vi "Frequency_Response_Data_Smoothing_Shifting.vi"(0 "smoothing":bool, 1 "curveShifting":bool) -> ()   [LabVIEW 2012]
uses:
  <vilib>/Analysis/6fits.llb/Curve Fitting Criteria.ctl
  <vilib>/Analysis/6fits.llb/General Linear Fit Algorithm.ctl
  <vilib>/Analysis/NI_AALPro.lvlib
panel:
  in  "FG.FrequencyLists.FrequencyResponse_LimitLow.amplitude":dbl[](array[numeric])
  in  "FG.FrequencyLists.FrequencyResponse_LimitHigh.amplitude":dbl[](array[numeric])
  in  "Parameters.UUTResponseLevel.amplitude":dbl[](array[numeric])
  in  "Parameters.UUTResponseLevel.frequency":dbl[](array[numeric])
  in  "Parameters.RefAmplitude":dbl=0.357
  out "XY Graph 2":cluster{dbl[], dbl[]}[](graph)=[{[200.0, 212.0, 224.0, 236.0, 250.0, 265.0, 280.0, 300.0, 315.0, 335.0, 355.0, 375.0, 400.0, 425.0, 450.0, 475.0, 500.0, 530.0, 560.0, 600.0, 630.0, 670.0, 710.0, 750.0, 800.0, 850.0, 900.0, 950.0, 1000.0, 1060.0, 1120.0, 1180.0, 1250.0, 1320.0, 1400.0, 1500.0, 1600.0, 1700.0, 1800.0, 1900.0, 2000.0, 2120.0, 2240.0, 2360.0, 2500.0, 2650.0, 2800.0, 3000.0, 3150.0, 3350.0, 3750.0, 4000.0, 4250.0, 4500.0, 4750.0, 5000.0, 5300.0, 5600.0, 6000.0, 6300.0, 6700.0, 7100.0], [-7.2, -6.8, -6.3, -5.7, -5.9, -5.2, -5.2, -4.5, -4.4, -3.9, -3.4, -3.2, -2.9, -2.6, -2.4, -2.1, -1.9, -1.7, -1.5, -1.3, -1.3, -1.1, -0.8, -0.8, -0.7, -0.6, -0.3, -0.5, 0.0, -0.3, 0.0, 0.2, 0.2, 0.4, 0.8, 0.9, 1.5, 1.5, 1.6, 1.5, 1.4, 0.6, -0.5, -1.5, -1.6, -2.3, -2.5, -3.0, -2.7, -3.1, -4.1, -5.6, -4.3, -3.1, -2.0, -0.7, 0.0, -1.0, 0.0, 0.5, 0.9, 3.6]}, {[200.0, 212.0, 224.0, 236.0, 250.0, 265.0, 280.0, 300.0, 315.0, 335.0, 355.0, 375.0, 400.0, 425.0, 450.0, 475.0, 500.0, 530.0, 560.0, 600.0, 630.0, 670.0, 710.0, 750.0, 800.0, 850.0, 900.0, 950.0, 1000.0, 1060.0, 1120.0, 1180.0, 1250.0, 1320.0, 1400.0, 1500.0, 1600.0, 1700.0, 1800.0, 1900.0, 2000.0, 2120.0, 2240.0, 2360.0, 2500.0, 2650.0, 2800.0, 3000.0, 3150.0, 3350.0, 3750.0, 4000.0, 4250.0, 4500.0, 4750.0, 5000.0, 5300.0, 5600.0, 6000.0, 6300.0, 6700.0, 7100.0], [-1.1, -0.9, -0.8, -0.6, -0.4, -0.2, 0.0, 0.1, 0.3, 0.5, 0.7, 0.9, 1.0, 1.2, 1.3, 1.5, 1.6, 1.7, 1.9, 2.0, 2.2, 2.3, 2.5, 2.6, 2.8, 2.9, 3.0, 3.0, 3.0, 3.0, 3.1, 3.1, 3.2, 3.2, 3.3, 3.3, 3.4, 3.5, 3.5, 3.6, 3.6, 3.7, 3.8, 3.8, 3.9, 3.9, 4.0, 4.3, 4.7, 5.1, 5.5, 5.9, 6.2, 6.5, 6.8, 7.1, 7.4, 7.7, 8.0, 7.6, 7.2, 6.8]}, {[200.0, 212.0, 224.0, 236.0, 250.0, 265.0, 280.0, 300.0, 315.0, 335.0, 355.0, 375.0, 400.0, 425.0, 450.0, 475.0, 500.0, 530.0, 560.0, 600.0, 630.0, 670.0, 710.0, 750.0, 800.0, 850.0, 900.0, 950.0, 1000.0, 1060.0, 1120.0, 1180.0, 1250.0, 1320.0, 1400.0, 1500.0, 1600.0, 1700.0, 1800.0, 1900.0, 2000.0, 2120.0, 2240.0, 2360.0, 2500.0, 2650.0, 2800.0, 3000.0, 3150.0, 3350.0, 3750.0, 4000.0, 4250.0, 4500.0, 4750.0, 5000.0, 5300.0, 5600.0, 6000.0, 6300.0, 6700.0, 7100.0], [-12.1, -11.5, -10.9, -10.3, -9.7, -9.1, -8.5, -7.9, -7.3, -6.7, -6.1, -5.5, -5.0, -4.8, -4.7, -4.5, -4.4, -4.3, -4.1, -4.0, -3.8, -3.7, -3.5, -3.4, -3.2, -3.1, -3.0, -3.0, -3.0, -3.0, -3.0, -3.0, -3.0, -3.0, -3.0, -3.0, -3.0, -3.0, -3.0, -3.0, -3.0, -3.0, -3.0, -3.0, -3.0, -3.0, -3.0, -3.0, -3.0, -3.0, -3.0, -3.0, -3.0, -3.0, -3.0, -3.0, -3.0, -3.0, -3.0, -3.2, -3.4, -3.6]}, {[199.67341715670165, 211.21395804831343, 223.6398834792109, 236.91827495666882, 251.0357328679638, 265.996892987689, 281.82294298506883, 298.5501389312743, 316.2283218067368, 334.9194340084638, 354.69603585735297, 375.63982210550773, 397.84013844355104, 421.3924980079408, 446.39709788828463, 472.9573356346543, 501.1783257649011, 531.1654162719695, 563.0227051312137, 596.8515568077104, 632.7491189432191, 670.8070219208591, 711.1119966697486, 753.7490969501578, 798.8054485348823, 846.3740041392261, 896.5572983509842, 949.4712025604283, 1005.2486798902885, 1064.043540125737, 1126.0341946443743, 1191.4274113462093, 1260.4620695836447, 1333.4129150914612, 1410.594314916799, 1492.3640123491455, 1579.126881850313, 1671.3386839844277, 1769.50982034791, 1874.2090884994595, 1986.0674368900388, 2105.781688039848, 2234.1153513535733, 2371.8850498380257, 2519.936351237608, 2679.118589027189, 2850.2596824126886, 3034.140956331676, 3231.4719614539495, 3442.865294182133, 3668.8114166522637, 3909.6534767343846, 4165.562128033129, 4436.510349888317, 4722.248267375544, 5022.277971306764, 5335.8283382308855, 5661.829850434362, 5998.8894159417805, 6345.26518851645, 6698.841387660996, 7057.103118617942], [-6.65792244532346, -6.805075217908138, -6.694954533621337, -6.4014241964905665, -5.9867078721014835, -5.502234641802871, -4.989484556911629, -4.480834192917781, -4.000402203689442, -3.564894875677825, -3.184451682122225, -2.86349083725501, -2.6015548505066124, -2.394156080710522, -2.23362229030827, -2.1099421995544265, -2.0116110407215864, -1.9264761123053604, -1.842582333229369, -1.749017797050228, -1.636759285351931, -1.499476235935405, -1.3338989352742925, -1.139595038692343, -0.9186263930106383, -0.6752045532551799, -0.41534629936446726, -0.14652915289708227, 0.12265310626072844, 0.3828349231874647, 0.624223451218799, 0.8369430352399845, 1.0113796949782774, 1.1385256082953537, 1.2103235944797202, 1.2200115975391388, 1.1624671694930382, 1.0345519536649335, 0.8354561679748401, 0.5670430882316968, 0.23419353142577315, -0.15485086731731323, -0.5882549462370955, -1.0509038551327632, -1.5251194336044547, -1.9914149659351008, -2.4292499736703292, -2.8177850081983906, -3.1366364433300533, -3.366631267878519, -3.4905618782393444, -3.4939408709703432, -3.3657558353715027, -3.09922414606489, -2.69254775557457, -2.1496679869065165, -1.481020326128518, -0.7042892149500959, 0.15483715669758005, 1.0619120580818044, 1.972975425088389, 2.8337990676417735]}, {[200.0, 212.0, 224.0, 236.0, 250.0, 265.0, 280.0, 300.0, 315.0, 335.0, 355.0, 375.0, 400.0, 425.0, 450.0, 475.0, 500.0, 530.0, 560.0, 600.0, 630.0, 670.0, 710.0, 750.0, 800.0, 850.0, 900.0, 950.0, 1000.0, 1060.0, 1120.0, 1180.0, 1250.0, 1320.0, 1400.0, 1500.0, 1600.0, 1700.0, 1800.0, 1900.0, 2000.0, 2120.0, 2240.0, 2360.0, 2500.0, 2650.0, 2800.0, 3000.0, 3150.0, 3350.0, 3750.0, 4000.0, 4250.0, 4500.0, 4750.0, 5000.0, 5300.0, 5600.0, 6000.0, 6300.0, 6700.0, 7100.0], [-6.205157643136481, -6.020933720665548, -5.839820813498944, -5.661789291037467, -5.457941067757162, -5.244089074811557, -5.034895452852371, -4.763119446794431, -4.564576452219682, -4.306798833759117, -4.056840237791941, -3.814571221558727, -3.52235316631936, -3.2417019360107107, -2.9723725806568284, -2.7141230359897723, -2.4667141079946853, -2.1838004428542828, -1.9157540870861651, -1.5808002758181445, -1.3459098706888752, -1.0537598512323598, -0.7848342367946678, -0.5382573519035433, -0.2601588393533418, -0.014004002741201994, 0.20180170104589448, 0.3888108475350209, 0.548534539225186, 0.7062532479133133, 0.82925925924909, 0.919933372917582, 0.9879189654908209, 1.0185369247443874, 1.012085590476093, 0.9488508818517398, 0.8325442205002949, 0.6714424338723249, 0.4732695619414947, 0.24521268305773286, -0.00606226019973688, -0.3296005042348227, -0.668009124585811, -1.012545565513891, -1.4118853982716553, -1.8249503288668656, -2.211639742848497, -2.6702265839668047, -2.9619969125583223, -3.271384677495506, -3.591217499070522, -3.5837982599559837, -3.4242772734673714, -3.126780435781683, -2.7106446731240332, -2.198872448299305, -1.493935993511684, -0.7316998047271994, 0.3027856705332539, 1.048904055149677, 1.9656754194686528, 2.7927851528351084]}, {[200.0, 212.0, 224.0, 236.0, 250.0, 265.0, 280.0, 300.0, 315.0, 335.0, 355.0, 375.0, 400.0, 425.0, 450.0, 475.0, 500.0, 530.0, 560.0, 600.0, 630.0, 670.0, 710.0, 750.0, 800.0, 850.0, 900.0, 950.0, 1000.0, 1060.0, 1120.0, 1180.0, 1250.0, 1320.0, 1400.0, 1500.0, 1600.0, 1700.0, 1800.0, 1900.0, 2000.0, 2120.0, 2240.0, 2360.0, 2500.0, 2650.0, 2800.0, 3000.0, 3150.0, 3350.0, 3750.0, 4000.0, 4250.0, 4500.0, 4750.0, 5000.0, 5300.0, 5600.0, 6000.0, 6300.0, 6700.0, 7100.0], [-4.819515580060011, -4.635291657589078, -4.454178750422474, -4.276147227960997, -4.0722990046806915, -3.8584470117350866, -3.649253389775901, -3.3774773837179612, -3.178934389143212, -2.9211567706826473, -2.671198174715471, -2.4289291584822568, -2.13671110324289, -1.8560598729342406, -1.5867305175803583, -1.3284809729133022, -1.0810720449182152, -0.7981583797778127, -0.530112024009695, -0.19515821274167444, 0.039732192387594845, 0.33188221184411026, 0.6008078262818023, 0.8473847111729268, 1.1254832237231283, 1.371638060335268, 1.5874437641223647, 1.774452910611491, 1.934176602301656, 2.0918953109897833, 2.2149013223255603, 2.305575435994052, 2.3735610285672912, 2.4041789878208575, 2.397727653552563, 2.33449294492821, 2.218186283576765, 2.057084496948795, 1.858911625017965, 1.630854746134203, 1.3795798028767332, 1.0560415588416474, 0.7176329384906591, 0.373096497562579, -0.02624333519518518, -0.4393082657903955, -0.8259976797720268, -1.2845845208903346, -1.5763548494818522, -1.8857426144190361, -2.205575435994052, -2.1981561968795136, -2.0386352103909013, -1.7411383727052128, -1.3250026100475631, -0.8132303852228349, -0.10829393043521396, 0.6539422583492707, 1.688427733609724, 2.434546118226147, 3.351317482545123, 4.1784272159115785]}, {[100.0, 109.75, 120.451, 132.194, 145.083, 151.991, 159.229, 166.81, 174.753, 183.074, 191.791, 200.924, 210.491, 220.514, 231.013, 242.013, 253.537, 265.609, 278.256, 291.506, 305.386, 319.927, 335.161, 351.12, 367.839, 385.354, 403.702, 422.925, 443.063, 464.16, 486.261, 509.415, 533.671, 559.082, 585.703, 613.592, 642.808, 673.416, 705.481, 739.073, 774.265, 800.0, 811.132, 849.755, 890.216, 932.604, 977.011, 1000.0, 1023.53, 1072.27, 1123.33, 1176.81, 1200.0, 1232.85, 1291.55, 1353.05, 1417.48, 1484.97, 1500.0, 1555.68, 1629.75, 1707.35, 1788.65, 1873.82, 1963.04, 2056.51, 2154.44, 2257.02, 2364.49, 2477.08, 2595.03, 2718.59, 2848.04, 3000.0, 3125.72, 3274.55, 3430.47, 3593.81, 3764.94, 3944.21, 4132.01, 4328.76, 4534.88, 4750.81, 4977.02, 5214.01, 5462.28, 5722.37, 5994.84, 6280.29, 6579.33, 6892.61, 7220.81, 7564.63, 7924.83, 8302.18, 8697.49, 9111.63, 9545.48, 10000.0], [-12.5364598, -11.56399749, -10.71471488, -9.746106214, -8.932955816, -8.623519657, -8.202587644, -7.922776867, -7.459536057, -7.176896594, -6.767276149, -6.621141225, -6.163309576, -5.821858782, -5.565218706, -5.250113325, -4.88377693, -4.520980439, -4.128279329, -3.967779369, -3.439989214, -3.306802936, -3.022521512, -2.752079811, -2.67908037, -2.443687791, -2.19237044, -1.901898825, -1.645061848, -1.465411195, -1.328138675, -1.105365215, -0.93406896, -0.833701191, -0.58134861, -0.589684154, -0.389469189, -0.238374704, -0.082247804, -0.090033008, 0.030472777, 0.095630841, 0.188416686, 0.381096316, 0.352662557, 0.435375392, 0.330187127, 0.014538785, 0.49282774, 0.501267915, 0.646232832, 0.629987721, 0.631156515, 0.759233712, 0.817208809, 0.802986805, 0.856497026, 0.822189906, 0.879343869, 1.092334977, 1.083390244, 1.421459455, 1.422692428, 1.698786337, 1.643719715, 1.814571472, 2.308763915, 2.175171376, 1.8065676, 1.599622752, 1.045092499, 0.713123986, 0.374411241, 0.485911234, 0.397252935, 0.522621826, -0.602007918, -0.888162805, -0.310495703, 0.206080955, 0.901098591, 0.46502272, 0.174905366, 2.086975243, 3.413118757, 3.408819036, 3.043681804, 3.15649832, 2.281101071, -0.176361996, 0.33128943, 0.491323472, -0.711805785, -0.350241622, -0.65271294, -0.54228727, -1.727402173, -1.413133064, -3.760874502, -3.709952127]}]
  out "max value":dbl=0.5912174990705221
  out "min value":dbl=2.180066627082418
  out "ShiftCurveBy":dbl=1.38564206307647
  out "XY Graph":cluster{dbl[], dbl[]}[](graph)=[{[200.0, 212.0, 224.0, 236.0, 250.0, 265.0, 280.0, 300.0, 315.0, 335.0, 355.0, 375.0, 400.0, 425.0, 450.0, 475.0, 500.0, 530.0, 560.0, 600.0, 630.0, 670.0, 710.0, 750.0, 800.0, 850.0, 900.0, 950.0, 1000.0, 1060.0, 1120.0, 1180.0, 1250.0, 1320.0, 1400.0, 1500.0, 1600.0, 1700.0, 1800.0, 1900.0, 2000.0, 2120.0, 2240.0, 2360.0, 2500.0, 2650.0, 2800.0, 3000.0, 3150.0, 3350.0, 3750.0, 4000.0, 4250.0, 4500.0, 4750.0, 5000.0, 5300.0, 5600.0, 6000.0, 6300.0, 6700.0, 7100.0], [-7.2, -6.8, -6.3, -5.7, -5.9, -5.2, -5.2, -4.5, -4.4, -3.9, -3.4, -3.2, -2.9, -2.6, -2.4, -2.1, -1.9, -1.7, -1.5, -1.3, -1.3, -1.1, -0.8, -0.8, -0.7, -0.6, -0.3, -0.5, 0.0, -0.3, 0.0, 0.2, 0.2, 0.4, 0.8, 0.9, 1.5, 1.5, 1.6, 1.5, 1.4, 0.6, -0.5, -1.5, -1.6, -2.3, -2.5, -3.0, -2.7, -3.1, -4.1, -5.6, -4.3, -3.1, -2.0, -0.7, 0.0, -1.0, 0.0, 0.5, 0.9, 3.6]}, {[200.0, 212.0, 224.0, 236.0, 250.0, 265.0, 280.0, 300.0, 315.0, 335.0, 355.0, 375.0, 400.0, 425.0, 450.0, 475.0, 500.0, 530.0, 560.0, 600.0, 630.0, 670.0, 710.0, 750.0, 800.0, 850.0, 900.0, 950.0, 1000.0, 1060.0, 1120.0, 1180.0, 1250.0, 1320.0, 1400.0, 1500.0, 1600.0, 1700.0, 1800.0, 1900.0, 2000.0, 2120.0, 2240.0, 2360.0, 2500.0, 2650.0, 2800.0, 3000.0, 3150.0, 3350.0, 3750.0, 4000.0, 4250.0, 4500.0, 4750.0, 5000.0, 5300.0, 5600.0, 6000.0, 6300.0, 6700.0, 7100.0], [-1.1, -0.9, -0.8, -0.6, -0.4, -0.2, 0.0, 0.1, 0.3, 0.5, 0.7, 0.9, 1.0, 1.2, 1.3, 1.5, 1.6, 1.7, 1.9, 2.0, 2.2, 2.3, 2.5, 2.6, 2.8, 2.9, 3.0, 3.0, 3.0, 3.0, 3.1, 3.1, 3.2, 3.2, 3.3, 3.3, 3.4, 3.5, 3.5, 3.6, 3.6, 3.7, 3.8, 3.8, 3.9, 3.9, 4.0, 4.3, 4.7, 5.1, 5.5, 5.9, 6.2, 6.5, 6.8, 7.1, 7.4, 7.7, 8.0, 7.6, 7.2, 6.8]}, {[200.0, 212.0, 224.0, 236.0, 250.0, 265.0, 280.0, 300.0, 315.0, 335.0, 355.0, 375.0, 400.0, 425.0, 450.0, 475.0, 500.0, 530.0, 560.0, 600.0, 630.0, 670.0, 710.0, 750.0, 800.0, 850.0, 900.0, 950.0, 1000.0, 1060.0, 1120.0, 1180.0, 1250.0, 1320.0, 1400.0, 1500.0, 1600.0, 1700.0, 1800.0, 1900.0, 2000.0, 2120.0, 2240.0, 2360.0, 2500.0, 2650.0, 2800.0, 3000.0, 3150.0, 3350.0, 3750.0, 4000.0, 4250.0, 4500.0, 4750.0, 5000.0, 5300.0, 5600.0, 6000.0, 6300.0, 6700.0, 7100.0], [-12.1, -11.5, -10.9, -10.3, -9.7, -9.1, -8.5, -7.9, -7.3, -6.7, -6.1, -5.5, -5.0, -4.8, -4.7, -4.5, -4.4, -4.3, -4.1, -4.0, -3.8, -3.7, -3.5, -3.4, -3.2, -3.1, -3.0, -3.0, -3.0, -3.0, -3.0, -3.0, -3.0, -3.0, -3.0, -3.0, -3.0, -3.0, -3.0, -3.0, -3.0, -3.0, -3.0, -3.0, -3.0, -3.0, -3.0, -3.0, -3.0, -3.0, -3.0, -3.0, -3.0, -3.0, -3.0, -3.0, -3.0, -3.0, -3.0, -3.2, -3.4, -3.6]}, {[199.67341715670165, 211.21395804831343, 223.6398834792109, 236.91827495666882, 251.0357328679638, 265.996892987689, 281.82294298506883, 298.5501389312743, 316.2283218067368, 334.9194340084638, 354.69603585735297, 375.63982210550773, 397.84013844355104, 421.3924980079408, 446.39709788828463, 472.9573356346543, 501.1783257649011, 531.1654162719695, 563.0227051312137, 596.8515568077104, 632.7491189432191, 670.8070219208591, 711.1119966697486, 753.7490969501578, 798.8054485348823, 846.3740041392261, 896.5572983509842, 949.4712025604283, 1005.2486798902885, 1064.043540125737, 1126.0341946443743, 1191.4274113462093, 1260.4620695836447, 1333.4129150914612, 1410.594314916799, 1492.3640123491455, 1579.126881850313, 1671.3386839844277, 1769.50982034791, 1874.2090884994595, 1986.0674368900388, 2105.781688039848, 2234.1153513535733, 2371.8850498380257, 2519.936351237608, 2679.118589027189, 2850.2596824126886, 3034.140956331676, 3231.4719614539495, 3442.865294182133, 3668.8114166522637, 3909.6534767343846, 4165.562128033129, 4436.510349888317, 4722.248267375544, 5022.277971306764, 5335.8283382308855, 5661.829850434362, 5998.8894159417805, 6345.26518851645, 6698.841387660996, 7057.103118617942], [-6.65792244532346, -6.805075217908138, -6.694954533621337, -6.4014241964905665, -5.9867078721014835, -5.502234641802871, -4.989484556911629, -4.480834192917781, -4.000402203689442, -3.564894875677825, -3.184451682122225, -2.86349083725501, -2.6015548505066124, -2.394156080710522, -2.23362229030827, -2.1099421995544265, -2.0116110407215864, -1.9264761123053604, -1.842582333229369, -1.749017797050228, -1.636759285351931, -1.499476235935405, -1.3338989352742925, -1.139595038692343, -0.9186263930106383, -0.6752045532551799, -0.41534629936446726, -0.14652915289708227, 0.12265310626072844, 0.3828349231874647, 0.624223451218799, 0.8369430352399845, 1.0113796949782774, 1.1385256082953537, 1.2103235944797202, 1.2200115975391388, 1.1624671694930382, 1.0345519536649335, 0.8354561679748401, 0.5670430882316968, 0.23419353142577315, -0.15485086731731323, -0.5882549462370955, -1.0509038551327632, -1.5251194336044547, -1.9914149659351008, -2.4292499736703292, -2.8177850081983906, -3.1366364433300533, -3.366631267878519, -3.4905618782393444, -3.4939408709703432, -3.3657558353715027, -3.09922414606489, -2.69254775557457, -2.1496679869065165, -1.481020326128518, -0.7042892149500959, 0.15483715669758005, 1.0619120580818044, 1.972975425088389, 2.8337990676417735]}, {[200.0, 212.0, 224.0, 236.0, 250.0, 265.0, 280.0, 300.0, 315.0, 335.0, 355.0, 375.0, 400.0, 425.0, 450.0, 475.0, 500.0, 530.0, 560.0, 600.0, 630.0, 670.0, 710.0, 750.0, 800.0, 850.0, 900.0, 950.0, 1000.0, 1060.0, 1120.0, 1180.0, 1250.0, 1320.0, 1400.0, 1500.0, 1600.0, 1700.0, 1800.0, 1900.0, 2000.0, 2120.0, 2240.0, 2360.0, 2500.0, 2650.0, 2800.0, 3000.0, 3150.0, 3350.0, 3750.0, 4000.0, 4250.0, 4500.0, 4750.0, 5000.0, 5300.0, 5600.0, 6000.0, 6300.0, 6700.0, 7100.0], [-6.205157643136481, -6.020933720665548, -5.839820813498944, -5.661789291037467, -5.457941067757162, -5.244089074811557, -5.034895452852371, -4.763119446794431, -4.564576452219682, -4.306798833759117, -4.056840237791941, -3.814571221558727, -3.52235316631936, -3.2417019360107107, -2.9723725806568284, -2.7141230359897723, -2.4667141079946853, -2.1838004428542828, -1.9157540870861651, -1.5808002758181445, -1.3459098706888752, -1.0537598512323598, -0.7848342367946678, -0.5382573519035433, -0.2601588393533418, -0.014004002741201994, 0.20180170104589448, 0.3888108475350209, 0.548534539225186, 0.7062532479133133, 0.82925925924909, 0.919933372917582, 0.9879189654908209, 1.0185369247443874, 1.012085590476093, 0.9488508818517398, 0.8325442205002949, 0.6714424338723249, 0.4732695619414947, 0.24521268305773286, -0.00606226019973688, -0.3296005042348227, -0.668009124585811, -1.012545565513891, -1.4118853982716553, -1.8249503288668656, -2.211639742848497, -2.6702265839668047, -2.9619969125583223, -3.271384677495506, -3.591217499070522, -3.5837982599559837, -3.4242772734673714, -3.126780435781683, -2.7106446731240332, -2.198872448299305, -1.493935993511684, -0.7316998047271994, 0.3027856705332539, 1.048904055149677, 1.9656754194686528, 2.7927851528351084]}, {[200.0, 212.0, 224.0, 236.0, 250.0, 265.0, 280.0, 300.0, 315.0, 335.0, 355.0, 375.0, 400.0, 425.0, 450.0, 475.0, 500.0, 530.0, 560.0, 600.0, 630.0, 670.0, 710.0, 750.0, 800.0, 850.0, 900.0, 950.0, 1000.0, 1060.0, 1120.0, 1180.0, 1250.0, 1320.0, 1400.0, 1500.0, 1600.0, 1700.0, 1800.0, 1900.0, 2000.0, 2120.0, 2240.0, 2360.0, 2500.0, 2650.0, 2800.0, 3000.0, 3150.0, 3350.0, 3750.0, 4000.0, 4250.0, 4500.0, 4750.0, 5000.0, 5300.0, 5600.0, 6000.0, 6300.0, 6700.0, 7100.0], [-4.819515580060011, -4.635291657589078, -4.454178750422474, -4.276147227960997, -4.0722990046806915, -3.8584470117350866, -3.649253389775901, -3.3774773837179612, -3.178934389143212, -2.9211567706826473, -2.671198174715471, -2.4289291584822568, -2.13671110324289, -1.8560598729342406, -1.5867305175803583, -1.3284809729133022, -1.0810720449182152, -0.7981583797778127, -0.530112024009695, -0.19515821274167444, 0.039732192387594845, 0.33188221184411026, 0.6008078262818023, 0.8473847111729268, 1.1254832237231283, 1.371638060335268, 1.5874437641223647, 1.774452910611491, 1.934176602301656, 2.0918953109897833, 2.2149013223255603, 2.305575435994052, 2.3735610285672912, 2.4041789878208575, 2.397727653552563, 2.33449294492821, 2.218186283576765, 2.057084496948795, 1.858911625017965, 1.630854746134203, 1.3795798028767332, 1.0560415588416474, 0.7176329384906591, 0.373096497562579, -0.02624333519518518, -0.4393082657903955, -0.8259976797720268, -1.2845845208903346, -1.5763548494818522, -1.8857426144190361, -2.205575435994052, -2.1981561968795136, -2.0386352103909013, -1.7411383727052128, -1.3250026100475631, -0.8132303852228349, -0.10829393043521396, 0.6539422583492707, 1.688427733609724, 2.434546118226147, 3.351317482545123, 4.1784272159115785]}, {[100.0, 109.75, 120.451, 132.194, 145.083, 151.991, 159.229, 166.81, 174.753, 183.074, 191.791, 200.924, 210.491, 220.514, 231.013, 242.013, 253.537, 265.609, 278.256, 291.506, 305.386, 319.927, 335.161, 351.12, 367.839, 385.354, 403.702, 422.925, 443.063, 464.16, 486.261, 509.415, 533.671, 559.082, 585.703, 613.592, 642.808, 673.416, 705.481, 739.073, 774.265, 800.0, 811.132, 849.755, 890.216, 932.604, 977.011, 1000.0, 1023.53, 1072.27, 1123.33, 1176.81, 1200.0, 1232.85, 1291.55, 1353.05, 1417.48, 1484.97, 1500.0, 1555.68, 1629.75, 1707.35, 1788.65, 1873.82, 1963.04, 2056.51, 2154.44, 2257.02, 2364.49, 2477.08, 2595.03, 2718.59, 2848.04, 3000.0, 3125.72, 3274.55, 3430.47, 3593.81, 3764.94, 3944.21, 4132.01, 4328.76, 4534.88, 4750.81, 4977.02, 5214.01, 5462.28, 5722.37, 5994.84, 6280.29, 6579.33, 6892.61, 7220.81, 7564.63, 7924.83, 8302.18, 8697.49, 9111.63, 9545.48, 10000.0], [-12.5364598, -11.56399749, -10.71471488, -9.746106214, -8.932955816, -8.623519657, -8.202587644, -7.922776867, -7.459536057, -7.176896594, -6.767276149, -6.621141225, -6.163309576, -5.821858782, -5.565218706, -5.250113325, -4.88377693, -4.520980439, -4.128279329, -3.967779369, -3.439989214, -3.306802936, -3.022521512, -2.752079811, -2.67908037, -2.443687791, -2.19237044, -1.901898825, -1.645061848, -1.465411195, -1.328138675, -1.105365215, -0.93406896, -0.833701191, -0.58134861, -0.589684154, -0.389469189, -0.238374704, -0.082247804, -0.090033008, 0.030472777, 0.095630841, 0.188416686, 0.381096316, 0.352662557, 0.435375392, 0.330187127, 0.014538785, 0.49282774, 0.501267915, 0.646232832, 0.629987721, 0.631156515, 0.759233712, 0.817208809, 0.802986805, 0.856497026, 0.822189906, 0.879343869, 1.092334977, 1.083390244, 1.421459455, 1.422692428, 1.698786337, 1.643719715, 1.814571472, 2.308763915, 2.175171376, 1.8065676, 1.599622752, 1.045092499, 0.713123986, 0.374411241, 0.485911234, 0.397252935, 0.522621826, -0.602007918, -0.888162805, -0.310495703, 0.206080955, 0.901098591, 0.46502272, 0.174905366, 2.086975243, 3.413118757, 3.408819036, 3.043681804, 3.15649832, 2.281101071, -0.176361996, 0.33128943, 0.491323472, -0.711805785, -0.350241622, -0.65271294, -0.54228727, -1.727402173, -1.413133064, -3.760874502, -3.709952127]}]
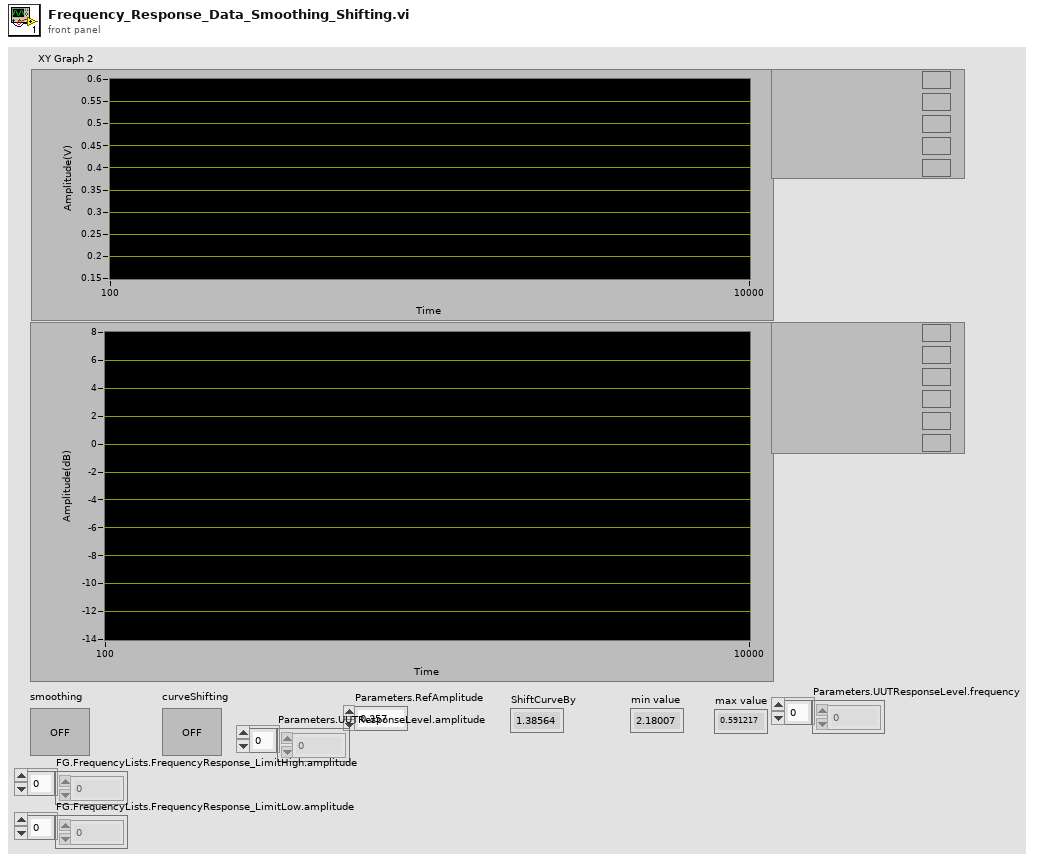
[diagram p1: front panel]
types:
  T1 = cluster{"Parameters.UUTResponseLevel.frequency":dbl[], dbl[]}
  T2 = cluster{"Parameters.UUTResponseLevel.frequency":dbl[], "FG.FrequencyLists.FrequencyResponse_LimitHigh.amplitude":dbl[]}
  T3 = cluster{"Parameters.UUTResponseLevel.frequency":dbl[], "FG.FrequencyLists.FrequencyResponse_LimitLow.amplitude":dbl[]}
  T4 = typedef "NI_AALPro.lvlib/General Linear Fit Algorithm.ctl" = u16
  T5 = typedef "NI_AALPro.lvlib/Curve Fitting Criteria.ctl" = u16
  T6 = cluster{"Parameters.UUTResponseLevel.frequency":dbl[], "Best Polynomial Fit":dbl[]}
  T7 = cluster{"Parameters.UUTResponseLevel.frequency":dbl[], dbl[]}[]
  T8 = cluster{"Parameters.UUTResponseLevel.frequency":dbl[], "Best Polynomial Fit":dbl[]}[]
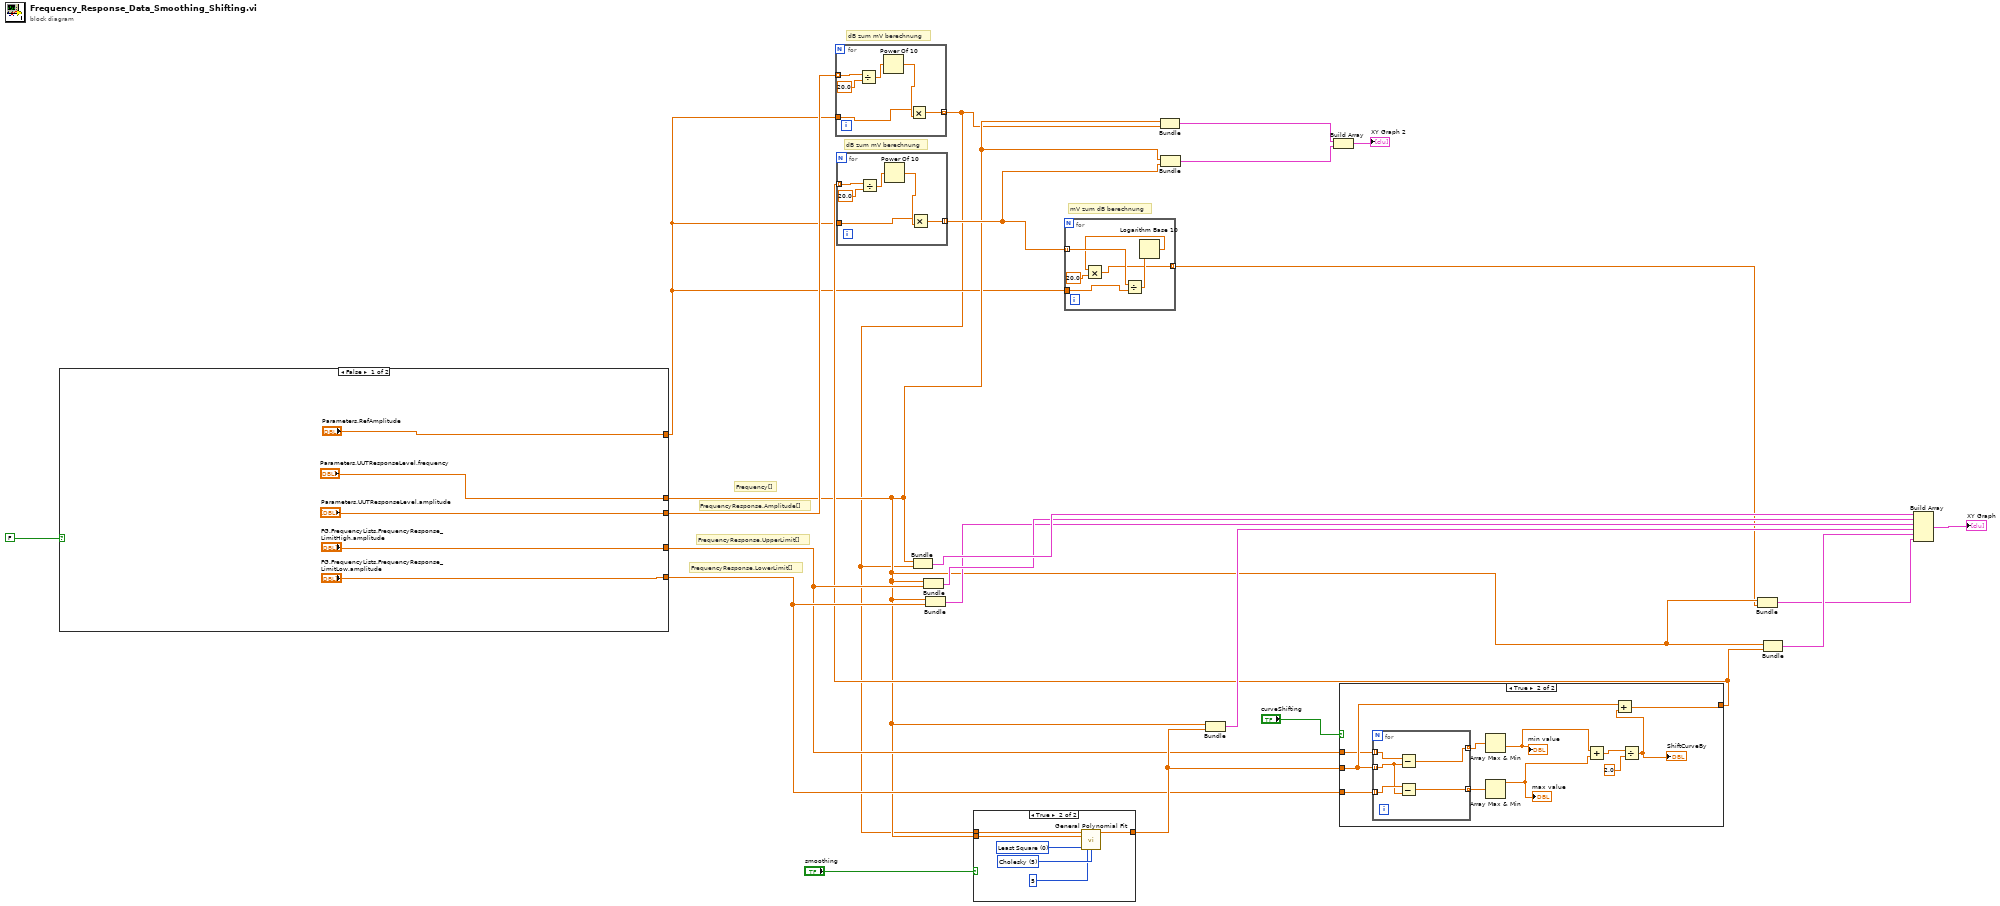
[diagram p0: block diagram]
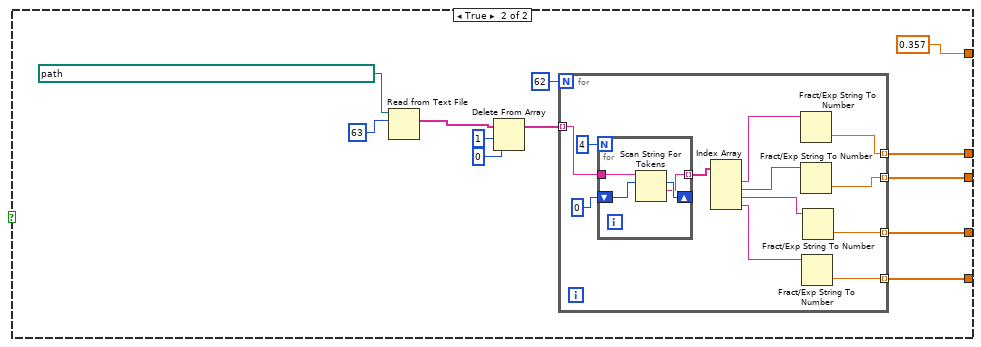
[diagram p2: hidden frame]
diagram:
  # "mV zum dB berechnung"
  # "dB zum mV berechnung"
  # "dB zum mV berechnung"
  # "FrequencyResponse.LowerLimit[]"
  # "FrequencyResponse.UpperLimit[]"
  # "FrequencyResponse.Amplitude[]"
  # "Frequency[]"
  n1 = case shown="False" FALSE {
    tunnel: ["FG.FrequencyLists.FrequencyResponse_LimitLow.amplitude" w33] -> w16
    tunnel: ["FG.FrequencyLists.FrequencyResponse_LimitHigh.amplitude" w32] -> w15
    tunnel: ["Parameters.UUTResponseLevel.amplitude" w31] -> w12
    tunnel: ["Parameters.UUTResponseLevel.frequency" w30] -> w6
    tunnel: ["Parameters.RefAmplitude" 0.357 ("Parameters.RefAmplitude")] -> w2
    frame False {
    }
    frame True {
      n2 = Read from Text File(file (use dialog)=path "C:/Users/vr.ext/Desktop/Smoothing FG/SVT_Prüfstand_FG.txt", count=63) -> (text=w37:string[])  [unwired: 2 in, 3 out]
      n3 = Delete From Array(array=w37, length=1, index=0) -> (array with subset deleted=w34:string[])  [unwired: 1 out]
      n4 = for {
        N: 62 -> [_]
        tunnel: w34 -> [w50] mode=indexing
        tunnel: [w52] -> w30 mode=indexing
        tunnel: [w51] -> w31 mode=indexing
        tunnel: [w42] -> w32 mode=indexing
        tunnel: [w41] -> w33 mode=indexing
        n5 = for {
          N: 4 -> [_]
          tunnel: w50 -> [w55]
          shift-right: [w56] -> _
          shift-left: 0 ("count") -> [w54]
          tunnel: [w53] -> w48 mode=indexing
          n6 = Scan String For Tokens(8:w54, 9:w55) -> (1:w53:string, 2:w56:i32)  [unwired: 4 in, 2 out]
        }
        n7 = Index Array(array=w48) -> (element #1=w47:string, element #2=w46:string, element #3=w44:string, element #4=w43:string)  [unwired: 4 in]
        n8 = Fract/Exp String To Number(string=w47) -> (number=w52:dbl)  [unwired: 3 in, 1 out]
        n9 = Fract/Exp String To Number(string=w46) -> (number=w51:dbl)  [unwired: 3 in, 1 out]
        n10 = Fract/Exp String To Number(string=w43) -> (number=w41:dbl)  [unwired: 3 in, 1 out]
        n11 = Fract/Exp String To Number(string=w44) -> (number=w42:dbl)  [unwired: 3 in, 1 out]
      }
    }
  }
  n12 = for {
    tunnel: w12 -> [w62] mode=indexing
    tunnel: [w58] -> w1 mode=indexing
    tunnel: w2 -> [w57]
    n13 = Divide(x=w62, y=20.0) -> (x/y=w60:dbl)
    n14 = Power Of 10(x=w60) -> (10^x=w59:dbl)
    n15 = Multiply(x=w57, y=w59) -> (x*y=w58:dbl)
  }
  n16 = Bundle("Parameters.UUTResponseLevel.frequency"=w6, w1) -> (w21:T1)  [unwired: 1 in]
  n17 = Bundle("Parameters.UUTResponseLevel.frequency"=w6, "FG.FrequencyLists.FrequencyResponse_LimitHigh.amplitude"=w15) -> (w20:T2)  [unwired: 1 in]
  n18 = Bundle("Parameters.UUTResponseLevel.frequency"=w6, "FG.FrequencyLists.FrequencyResponse_LimitLow.amplitude"=w16) -> (w19:T3)  [unwired: 1 in]
  n19 = case shown="True" "smoothing" {
    tunnel: w1 -> [w63 w66]
    tunnel: w6 -> [_ w65]
    tunnel: [w63 w64] -> w18
    frame False {
    }
    frame True {
      w68 = T4 5 items=["SVD", "Givens", "Givens2", "Householder", "LU Decomposition", "Cholesky", "SVD for Rank Deficient H"] ("algorithm")
      w69 = T5 0 items=["Least Square", "Least Absolute Residual", "Bisquare"] ("method")
      n20 = call <vilib>:"General Polynomial Fit.vi"("Y"=w66, "polynomial order"=5, "X"=w65, "method"=w69, "algorithm"=w68) -> ("Best Polynomial Fit"=w64:dbl[])  [unwired: 7 in, 3 out]
    }
  }
  n21 = Bundle("Parameters.UUTResponseLevel.frequency"=w6, w1) -> (w10:T1)  [unwired: 1 in]
  n22 = Bundle("Parameters.UUTResponseLevel.frequency"=w6, "Best Polynomial Fit"=w18) -> (w22:T6)  [unwired: 1 in]
  n23 = case shown="True" "curveShifting" {
    tunnel: w18 -> [w70 w79]
    tunnel: [w70 w78] -> w9
    tunnel: w16 -> [_ w77]
    tunnel: w15 -> [_ w76]
    frame False {
    }
    frame True {
      n24 = for {
        tunnel: w76 -> [w86] mode=indexing
        tunnel: w79 -> [w83] mode=indexing
        tunnel: [w85] -> w81 mode=indexing
        tunnel: w77 -> [w84] mode=indexing
        tunnel: [w82] -> w80 mode=indexing
        n25 = Subtract(x=w86, y=w83) -> (x-y=w85:dbl)
        n26 = Subtract(x=w84, y=w83) -> (x-y=w82:dbl)
      }
      n27 = Array Max & Min(array=w81) -> (min value=w75:dbl)  [unwired: 3 out]
      "min value" <- w75
      n28 = Array Max & Min(array=w80) -> (max value=w74:dbl)  [unwired: 3 out]
      "max value" <- w74
      n29 = Add(x=w75, y=w74) -> (x+y=w73:dbl)
      n30 = Divide(x=w73, y=2.0) -> (x/y=w71:dbl)
      "ShiftCurveBy" <- w71
      n31 = Add(x=w79, y=w71) -> (x+y=w78:dbl[])
    }
  }
  n32 = for {
    tunnel: w9 -> [w92] mode=indexing
    tunnel: [w88] -> w7 mode=indexing
    tunnel: w2 -> [w87]
    n33 = Divide(x=w92, y=20.0) -> (x/y=w90:dbl)
    n34 = Power Of 10(x=w90) -> (10^x=w89:dbl)
    n35 = Multiply(x=w87, y=w89) -> (x*y=w88:dbl)
  }
  n36 = for {
    tunnel: w7 -> [w97] mode=indexing
    tunnel: [w94] -> w5 mode=indexing
    tunnel: w2 -> [w93]
    n37 = Divide(x=w97, y=w93) -> (x/y=w96:dbl)
    n38 = Logarithm Base 10(1:w96) -> (0:w95:dbl)
    n39 = Multiply(x=w95, y=20.0) -> (x*y=w94:dbl)
  }
  n40 = Bundle("Parameters.UUTResponseLevel.frequency"=w6, w7) -> (w8:T1)  [unwired: 1 in]
  n41 = Build Array(w10, w8) -> (→"XY Graph 2":T7)
  n42 = Bundle("Parameters.UUTResponseLevel.frequency"=w6, w5) -> (w4:T1)  [unwired: 1 in]
  n43 = Bundle("Parameters.UUTResponseLevel.frequency"=w6, "Best Polynomial Fit"=w9) -> (w17:T6)  [unwired: 1 in]
  n44 = Build Array(w21, w20, w19, w22, w17, w4) -> (→"XY Graph":T8)
